vi "Get_DO.vi"(8 "error in (no error)":errorcluster, 10 "PIN Number":i8, 11 "DI_DO in":refnum<class "DI_DO.lvclass">) -> (0 "error out":errorcluster, 2 "STATUS":string, 3 "DI_DO out":refnum<class "DI_DO.lvclass">)   [LabVIEW 2023, in "Driver_DI_DO.lvlib" / "DI_DO.lvclass"]
uses:
  DI_DO.lvclass
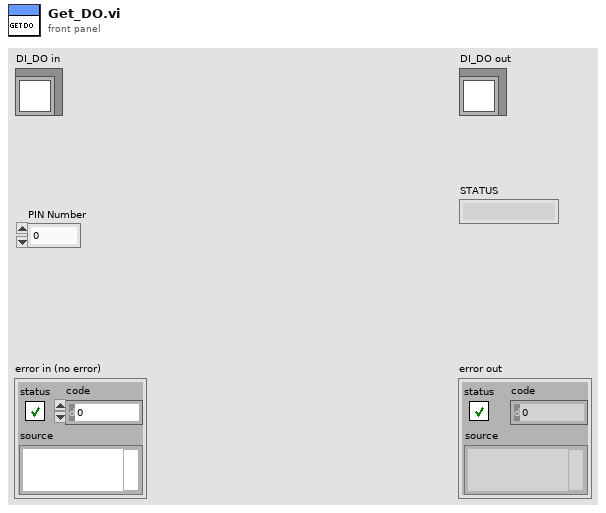
[diagram p1: front panel]
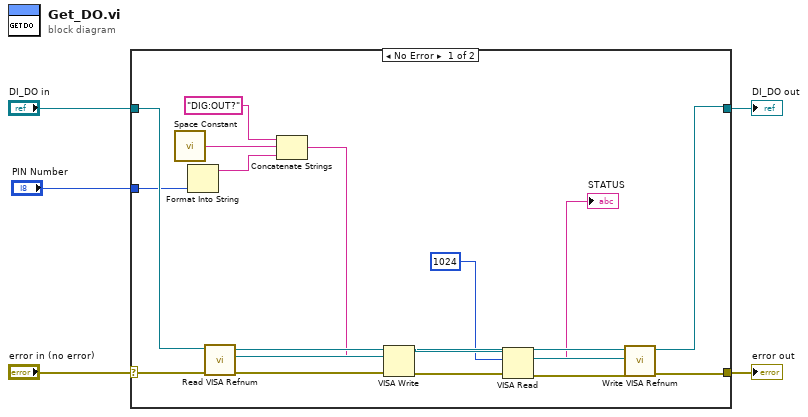
[diagram p0: block diagram]
diagram:
  n1 = case shown="No Error" "error in (no error)" {
    selector: "error in (no error)" -> [w21 w25]
    tunnel: [w16 w25] -> w4
    tunnel: [w15 w24] -> w2
    tunnel: "DI_DO in" -> [w20 w24]
    tunnel: "PIN Number" -> [w10 _]
    frame No Error {
      n2 = call <vilib>:"Space Constant.vi"() -> ("String"=w8:string)
      n3 = Format Into String(w10) -> (resulting string=w7:string)  [unwired: 3 in, 1 out]
      n4 = call-dynamic "Read VISA Refnum.vi"("error in (no error)"=w21, "Driver in"=w20) -> ("error out"=w18:errorcluster, "VISA Refnum"=w19:refnum<visa-resource-name>, "Driver out"=w14:refnum<class "DI_DO.lvclass">)  [unwired: 7 in]
      n5 = Concatenate Strings("DIG:OUT?" ("string"), w8, w7) -> (w6:string)
      n6 = VISA Write(VISA resource name=w19, write buffer=w6, error in (no error)=w18) -> (VISA resource name out=w22:refnum<visa-resource-name>, error out=w23:errorcluster)  [unwired: 1 out]
      n7 = VISA Read(VISA resource name=w22, byte count=u32 1024, error in (no error)=w23) -> (VISA resource name out=w12:refnum<visa-resource-name>, read buffer=→"STATUS":string, error out=w17:errorcluster)  [unwired: 1 out]
      n8 = call-dynamic "Write VISA Refnum.vi"("error in (no error)"=w17, "VISA Refnum"=w12, "Driver in"=w14) -> ("error out"=w16:errorcluster, "Driver out"=w15:refnum<class "DI_DO.lvclass">)  [unwired: 7 in]
    }
    frame Error {
    }
  }
  "error out" <- w4
  "DI_DO out" <- w2
